vi "Set Run Control.vi"(8 "error in (no error)":errorcluster, 10 "Run Control":T1, 11 "MSOX6004 in":refnum<class "MSOX6004.lvclass">) -> (0 "error out":errorcluster, 3 "MSOX6004 out":refnum<class "MSOX6004.lvclass">)   [LabVIEW 2018, in "MSOX6004.lvlib" / "MSOX6004.lvclass"]
doc: "This Override method is used to set the Oscope instrument running mode. The 'Run Control' control has 3 modes of operation: 0-Run (or continuous), 1 - Single, 2 - Stop."
uses:
  MSOX6004.lvclass
  PPLs/Oscilloscope/Parent/Oscilloscope.lvlibp/Custom Controls/Run Control.ctl
  MSOX6004.lvclass/MSOX6004.ctl
  <instrlib>/Keysight InfiniiVision/Keysight InfiniiVision.lvlib
  PPLs/Oscilloscope/Parent/Oscilloscope.lvlibp
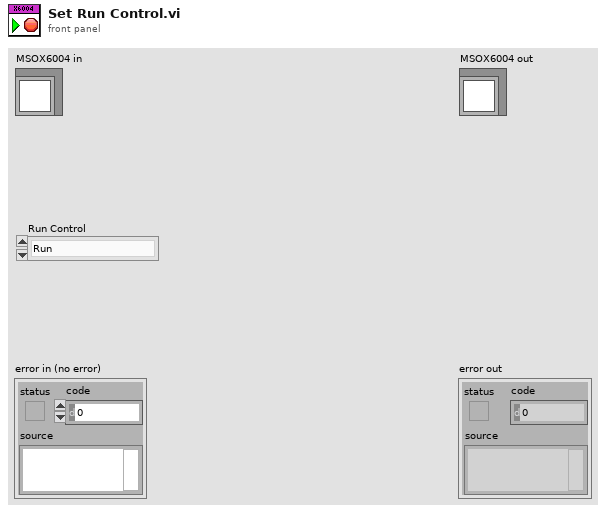
[diagram p1: front panel]
types:
  T1 = typedef "Oscilloscope.lvlibp/Run Control.ctl" = enum16{"Run", "Single", "Stop"}
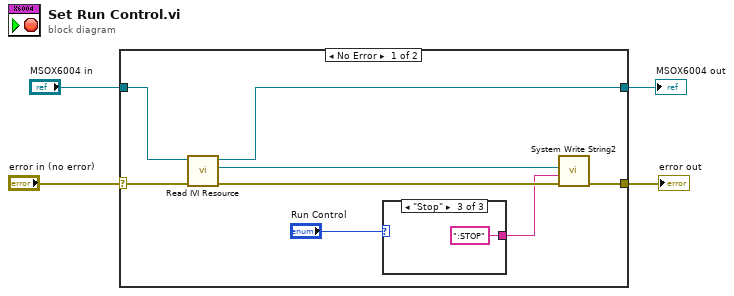
[diagram p0: block diagram]
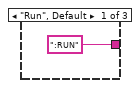
[diagram p2: hidden frame]
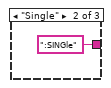
[diagram p3: hidden frame]
diagram:
  n1 = case shown="No Error" "error in (no error)" {
    selector: "error in (no error)" -> [w11 w17]
    tunnel: [w8 w17] -> w3
    tunnel: [w10 w16] -> w2
    tunnel: "MSOX6004 in" -> [w12 w16]
    frame No Error {
      n2 = call "Read IVI Resource.vi"("error in (no error)"=w11, "MSOX6004 in"=w12) -> ("error out"=w9:errorcluster, "IVI Resource"=w5:refnum<k15>, "MSOX6004 out"=w10:refnum<class "MSOX6004.lvclass">)  [unwired: 7 in]
      n3 = case shown="\"Stop\"" "Run Control" {
        tunnel: [":RUN" ":SINGle" ":STOP"] -> w6
        frame "Run", Default {
        }
        frame "Single" {
        }
        frame "Stop" {
        }
      }
      n4 = call <instrlib>:"System Write String2.vi"("error in (no error)"=w9, "Data"=w6, "instrument handle"=w5) -> ("error out"=w8:errorcluster)  [unwired: 7 in, 1 out]
    }
    frame Error {
    }
  }
  "error out" <- w3
  "MSOX6004 out" <- w2
